vi "ELVIS III v1.0 Write PWM.vi"(8 "error in (no error)":errorcluster, 9 "PWM Configuration In":T1, 10 "Channel":T2, 11 "myRIO Ref In":T3) -> (0 "error out":errorcluster, 2 "PWM Configuration Out":T1, 3 "myRIO Ref Out":T3)   [LabVIEW 2021]
uses:
  <vilib>/myRIO/Common/Instrument Driver Framework/Utilities/typedefs/myRIO v1.0 Reference.ctl
  <vilib>/myRIO/Common/Instrument Driver Framework/Utilities/typedefs/Generic FPGA Reference.ctl
  <vilib>/myRIO/Common/Instrument Driver Framework/myRIO v1.0/PWM/typedefs/PWM Channels Enum.ctl
  <vilib>/myRIO/Common/Instrument Driver Framework/myRIO v1.0/PWM/typedefs/PWM Configuration v1.0.ctl
  <vilib>/myRIO/Common/Instrument Driver Framework/ELVIS III v1.0/PWM/typedefs/ELVIS III PWM Channels FPGA Reference.ctl
  <vilib>/myRIO/Common/Instrument Driver Framework/Utilities/vis/Calculate Clock Settings.vi
  <vilib>/myRIO/Common/Instrument Driver Framework/Utilities/vis/Calculate TOP (Phase Correct Mode).vi
  <vilib>/myRIO/Common/Instrument Driver Framework/Utilities/vis/Calculate TOP (Normal Mode).vi
  <vilib>/myRIO/Common/Instrument Driver Framework/Utilities/vis/Calculate Frequency (Phase Correct Mode).vi
  <vilib>/myRIO/Common/Instrument Driver Framework/Utilities/vis/Calculate Frequency (Normal Mode).vi
  <vilib>/rvi/errors/niLvFpgaAdjustHostInterfaceError.vi
  <vilib>/rvi/interface/nirviReadWriteControl/nirviReadWriteControl.xnode
  NiFpgaLv.dll
  <vilib>/rvi/interface/Simulation/niFpgaSimulationCallBeginRW.vi
panel:
  # "This VI writes a value to each output compare register (OCCRA and OCCRB) for a particular PWM channel. The output compare values are used to define the duty cycles of the PWM outputs. Please see Block Diagram for details."
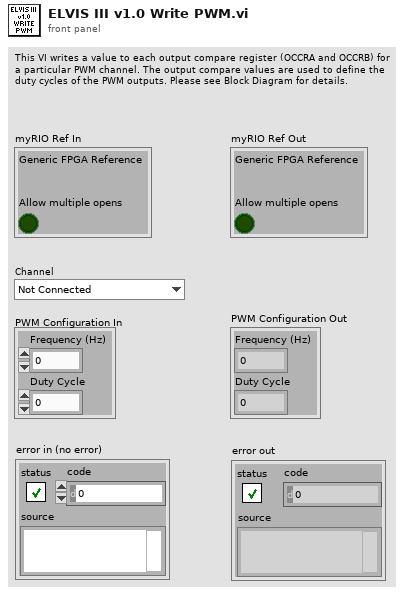
[diagram p1: front panel]
types:
  T1 = typedef "PWM Configuration v1.0.ctl" = cluster{"Frequency (Hz)":dbl, "Duty Cycle":dbl}
  T2 = typedef "PWM Channels Enum.ctl" = enum16{"Not Connected", "C/PWM0", "C/PWM1", "A/PWM0", "A/PWM1", "A/PWM2", "A/PWM3", "A/PWM4", "A/PWM5", "A/PWM6", "A/PWM7", "A/PWM8", "A/PWM9", "A/PWM10", "A/PWM11", "A/PWM12", "A/PWM13", "A/PWM14", "A/PWM15", "A/PWM16", "A/PWM17", "A/PWM18", "A/PWM19", "B/PWM0", "B/PWM1", "B/PWM2", "B/PWM3", "B/PWM4", "B/PWM5", "B/PWM6", "B/PWM7", "B/PWM8", "B/PWM9", "B/PWM10", "B/PWM11", "B/PWM12", "B/PWM13", "B/PWM14", "B/PWM15", "B/PWM16", "B/PWM17", "B/PWM18", "B/PWM19", "PWM/PWM0", "PWM/PWM1", "PWM/PWM2", "PWM/PWM3", "PWM/PWM4", "PWM/PWM5", "PWM/PWM6", "PWM/PWM7", "PWM/PWM8", "PWM/PWM9"}
  T3 = typedef "myRIO v1.0 Reference.ctl" = cluster{"Generic FPGA Reference":T4, "Allow multiple opens":bool}
  T4 = typedef "Generic FPGA Reference.ctl" = refnum<k20>
  T5 = typedef "ELVIS III PWM Channels FPGA Reference.ctl" = refnum<k20>
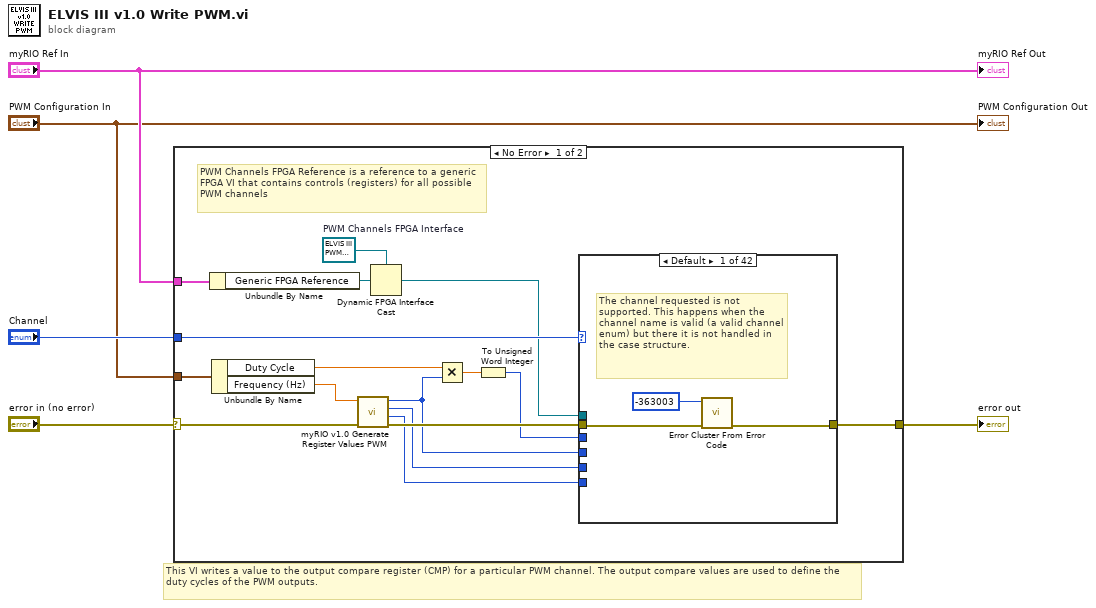
[diagram p0: block diagram]
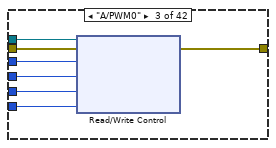
[diagram p3: hidden frame]
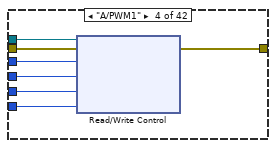
[diagram p4: hidden frame]
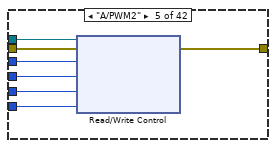
[diagram p5: hidden frame]
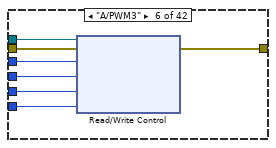
[diagram p6: hidden frame]
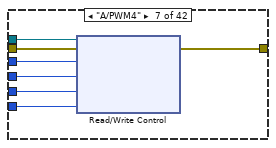
[diagram p7: hidden frame]
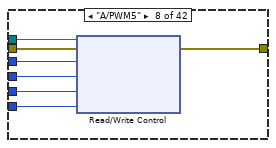
[diagram p8: hidden frame]
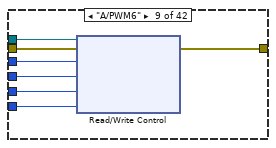
[diagram p9: hidden frame]
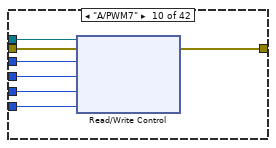
[diagram p10: hidden frame]
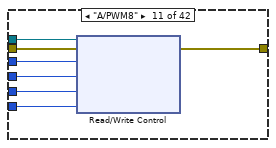
[diagram p11: hidden frame]
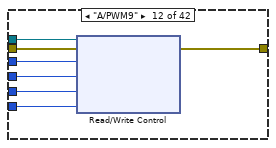
[diagram p12: hidden frame]
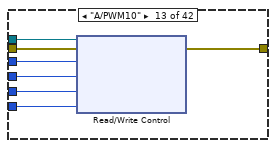
[diagram p13: hidden frame]
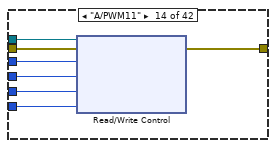
[diagram p14: hidden frame]
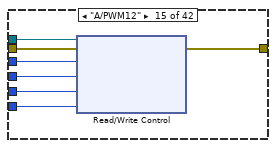
[diagram p15: hidden frame]
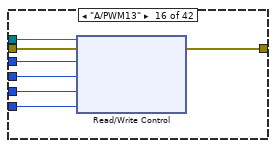
[diagram p16: hidden frame]
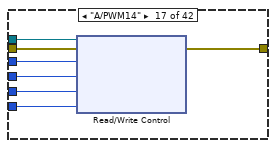
[diagram p17: hidden frame]
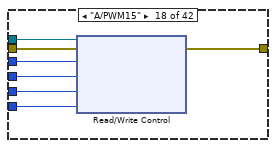
[diagram p18: hidden frame]
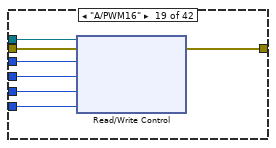
[diagram p19: hidden frame]
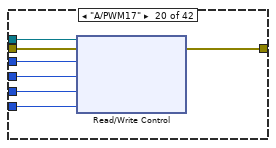
[diagram p20: hidden frame]
diagram:
  # "This VI writes a value to the output compare register (CMP) for a particular PWM channel. The output compare values are used to define the duty cycles of the PWM outputs."
  n1 = case shown="No Error" "error in (no error)" {
    selector: "error in (no error)" -> [w16 w306]
    tunnel: "myRIO Ref In" -> [w20 _]
    tunnel: [w6 w306] -> w4
    tunnel: "Channel" -> [w13 _]
    tunnel: "PWM Configuration In" -> [w15 _]
    frame No Error {
      w21 = T5 refnum  # PWM Channels FPGA Interface
      # "PWM Channels FPGA Reference is a reference to a generic FPGA VI that contains controls (registers) for all possible PWM channels"
      n2 = Unbundle By Name(w20) -> ("Generic FPGA Reference"=w19:T4)
      n3 = Unbundle By Name(w15) -> ("Duty Cycle"=w18:dbl, "Frequency (Hz)"=w14:dbl)
      n4 = call <vilib>:"myRIO v1.0 Generate Register Values PWM.vi"("error in (no error)"=w16, "Frequency (Hz)"=w14) -> ("error out"=w11:errorcluster, "PWM.CS"=w7:u8, "PWM.CNFG"=w8:u8, "PWM.MAX"=w9:u16)  [unwired: 5 in, 1 out]
      n5 = Dynamic FPGA Interface Cast(Session In=w21, Type=w19) -> (Session Out=w12:T5)
      n6 = Multiply(x=w18, y=w9) -> (x*y=w17:dbl)
      n7 = To Unsigned Word Integer(number=w17) -> (unsigned 16bit integer=w10:u16)
      n8 = case shown="Default" w13 {
        tunnel: w12 -> [_ _ w32 w39 w46 w53 w60 w67 w74 w81 w88 w95 w102 w109 w116 w123 w130 w137 w144 w151 w158 w165 w172 w179 w186 w193 w200 w207 w214 w221 w228 w235 w242 w249 w256 w263 w270 w277 w284 w291 w298 w305]
        tunnel: w11 -> [w23 w25 w31 w38 w45 w52 w59 w66 w73 w80 w87 w94 w101 w108 w115 w122 w129 w136 w143 w150 w157 w164 w171 w178 w185 w192 w199 w206 w213 w220 w227 w234 w241 w248 w255 w262 w269 w276 w283 w290 w297 w304]
        tunnel: w10 -> [_ _ w30 w37 w44 w51 w58 w65 w72 w79 w86 w93 w100 w107 w114 w121 w128 w135 w142 w149 w156 w163 w170 w177 w184 w191 w198 w205 w212 w219 w226 w233 w240 w247 w254 w261 w268 w275 w282 w289 w296 w303]
        tunnel: w9 -> [_ _ w29 w36 w43 w50 w57 w64 w71 w78 w85 w92 w99 w106 w113 w120 w127 w134 w141 w148 w155 w162 w169 w176 w183 w190 w197 w204 w211 w218 w225 w232 w239 w246 w253 w260 w267 w274 w281 w288 w295 w302]
        tunnel: w8 -> [_ _ w28 w35 w42 w49 w56 w63 w70 w77 w84 w91 w98 w105 w112 w119 w126 w133 w140 w147 w154 w161 w168 w175 w182 w189 w196 w203 w210 w217 w224 w231 w238 w245 w252 w259 w266 w273 w280 w287 w294 w301]
        tunnel: w7 -> [_ _ w27 w34 w41 w48 w55 w62 w69 w76 w83 w90 w97 w104 w111 w118 w125 w132 w139 w146 w153 w160 w167 w174 w181 w188 w195 w202 w209 w216 w223 w230 w237 w244 w251 w258 w265 w272 w279 w286 w293 w300]
        tunnel: [w22 w25 w26 w33 w40 w47 w54 w61 w68 w75 w82 w89 w96 w103 w110 w117 w124 w131 w138 w145 w152 w159 w166 w173 w180 w187 w194 w201 w208 w215 w222 w229 w236 w243 w250 w257 w264 w271 w278 w285 w292 w299] -> w6
        frame Default {
          # "The channel requested is not supported. This happens when the channel name is valid (a valid channel enum) but there it is not handled in the case structure."
          n9 = call <vilib>:"Error Cluster From Error Code.vi"("error in (no error)"=w23, "error code (0)"=-363003) -> ("error out"=w22:errorcluster)  [unwired: 7 in]
        }
        frame "Not Connected" {
        }
        frame "A/PWM0" {
          n10 = xnode "Read/Write Control"("FPGA VI Reference In"=w32, "error in"=w31, "PWM.A_0.CMP"=w30, "PWM.A_0.MAX"=w29, "PWM.A_0.CNFG"=w28, "PWM.A_0.CS"=w27) -> ("error out"=w26:errorcluster)  [unwired: 1 out]
        }
        frame "A/PWM1" {
          n11 = xnode "Read/Write Control"("FPGA VI Reference In"=w39, "error in"=w38, "PWM.A_1.CMP"=w37, "PWM.A_1.MAX"=w36, "PWM.A_1.CNFG"=w35, "PWM.A_1.CS"=w34) -> ("error out"=w33:errorcluster)  [unwired: 1 out]
        }
        frame "A/PWM2" {
          n12 = xnode "Read/Write Control"("FPGA VI Reference In"=w46, "error in"=w45, "PWM.A_2.CMP"=w44, "PWM.A_2.MAX"=w43, "PWM.A_2.CNFG"=w42, "PWM.A_2.CS"=w41) -> ("error out"=w40:errorcluster)  [unwired: 1 out]
        }
        frame "A/PWM3" {
          n13 = xnode "Read/Write Control"("FPGA VI Reference In"=w53, "error in"=w52, "PWM.A_3.CMP"=w51, "PWM.A_3.MAX"=w50, "PWM.A_3.CNFG"=w49, "PWM.A_3.CS"=w48) -> ("error out"=w47:errorcluster)  [unwired: 1 out]
        }
        frame "A/PWM4" {
          n14 = xnode "Read/Write Control"("FPGA VI Reference In"=w60, "error in"=w59, "PWM.A_4.CMP"=w58, "PWM.A_4.MAX"=w57, "PWM.A_4.CNFG"=w56, "PWM.A_4.CS"=w55) -> ("error out"=w54:errorcluster)  [unwired: 1 out]
        }
        frame "A/PWM5" {
          n15 = xnode "Read/Write Control"("FPGA VI Reference In"=w67, "error in"=w66, "PWM.A_5.CMP"=w65, "PWM.A_5.MAX"=w64, "PWM.A_5.CNFG"=w63, "PWM.A_5.CS"=w62) -> ("error out"=w61:errorcluster)  [unwired: 1 out]
        }
        frame "A/PWM6" {
          n16 = xnode "Read/Write Control"("FPGA VI Reference In"=w74, "error in"=w73, "PWM.A_6.CMP"=w72, "PWM.A_6.MAX"=w71, "PWM.A_6.CNFG"=w70, "PWM.A_6.CS"=w69) -> ("error out"=w68:errorcluster)  [unwired: 1 out]
        }
        frame "A/PWM7" {
          n17 = xnode "Read/Write Control"("FPGA VI Reference In"=w81, "error in"=w80, "PWM.A_7.CMP"=w79, "PWM.A_7.MAX"=w78, "PWM.A_7.CNFG"=w77, "PWM.A_7.CS"=w76) -> ("error out"=w75:errorcluster)  [unwired: 1 out]
        }
        frame "A/PWM8" {
          n18 = xnode "Read/Write Control"("FPGA VI Reference In"=w88, "error in"=w87, "PWM.A_8.CMP"=w86, "PWM.A_8.MAX"=w85, "PWM.A_8.CNFG"=w84, "PWM.A_8.CS"=w83) -> ("error out"=w82:errorcluster)  [unwired: 1 out]
        }
        frame "A/PWM9" {
          n19 = xnode "Read/Write Control"("FPGA VI Reference In"=w95, "error in"=w94, "PWM.A_9.CMP"=w93, "PWM.A_9.MAX"=w92, "PWM.A_9.CNFG"=w91, "PWM.A_9.CS"=w90) -> ("error out"=w89:errorcluster)  [unwired: 1 out]
        }
        frame "A/PWM10" {
          n20 = xnode "Read/Write Control"("FPGA VI Reference In"=w102, "error in"=w101, "PWM.A_10.CMP"=w100, "PWM.A_10.MAX"=w99, "PWM.A_10.CNFG"=w98, "PWM.A_10.CS"=w97) -> ("error out"=w96:errorcluster)  [unwired: 1 out]
        }
        frame "A/PWM11" {
          n21 = xnode "Read/Write Control"("FPGA VI Reference In"=w109, "error in"=w108, "PWM.A_11.CMP"=w107, "PWM.A_11.MAX"=w106, "PWM.A_11.CNFG"=w105, "PWM.A_11.CS"=w104) -> ("error out"=w103:errorcluster)  [unwired: 1 out]
        }
        frame "A/PWM12" {
          n22 = xnode "Read/Write Control"("FPGA VI Reference In"=w116, "error in"=w115, "PWM.A_12.CMP"=w114, "PWM.A_12.MAX"=w113, "PWM.A_12.CNFG"=w112, "PWM.A_12.CS"=w111) -> ("error out"=w110:errorcluster)  [unwired: 1 out]
        }
        frame "A/PWM13" {
          n23 = xnode "Read/Write Control"("FPGA VI Reference In"=w123, "error in"=w122, "PWM.A_13.CMP"=w121, "PWM.A_13.MAX"=w120, "PWM.A_13.CNFG"=w119, "PWM.A_13.CS"=w118) -> ("error out"=w117:errorcluster)  [unwired: 1 out]
        }
        frame "A/PWM14" {
          n24 = xnode "Read/Write Control"("FPGA VI Reference In"=w130, "error in"=w129, "PWM.A_14.CMP"=w128, "PWM.A_14.MAX"=w127, "PWM.A_14.CNFG"=w126, "PWM.A_14.CS"=w125) -> ("error out"=w124:errorcluster)  [unwired: 1 out]
        }
        frame "A/PWM15" {
          n25 = xnode "Read/Write Control"("FPGA VI Reference In"=w137, "error in"=w136, "PWM.A_15.CMP"=w135, "PWM.A_15.MAX"=w134, "PWM.A_15.CNFG"=w133, "PWM.A_15.CS"=w132) -> ("error out"=w131:errorcluster)  [unwired: 1 out]
        }
        frame "A/PWM16" {
          n26 = xnode "Read/Write Control"("FPGA VI Reference In"=w144, "error in"=w143, "PWM.A_16.CMP"=w142, "PWM.A_16.MAX"=w141, "PWM.A_16.CNFG"=w140, "PWM.A_16.CS"=w139) -> ("error out"=w138:errorcluster)  [unwired: 1 out]
        }
        frame "A/PWM17" {
          n27 = xnode "Read/Write Control"("FPGA VI Reference In"=w151, "error in"=w150, "PWM.A_17.CMP"=w149, "PWM.A_17.MAX"=w148, "PWM.A_17.CNFG"=w147, "PWM.A_17.CS"=w146) -> ("error out"=w145:errorcluster)  [unwired: 1 out]
        }
        frame "A/PWM18" {
          n28 = xnode "Read/Write Control"("FPGA VI Reference In"=w158, "error in"=w157, "PWM.A_18.CMP"=w156, "PWM.A_18.MAX"=w155, "PWM.A_18.CNFG"=w154, "PWM.A_18.CS"=w153) -> ("error out"=w152:errorcluster)  [unwired: 1 out]
        }
        frame "A/PWM19" {
          n29 = xnode "Read/Write Control"("FPGA VI Reference In"=w165, "error in"=w164, "PWM.A_19.CMP"=w163, "PWM.A_19.MAX"=w162, "PWM.A_19.CNFG"=w161, "PWM.A_19.CS"=w160) -> ("error out"=w159:errorcluster)  [unwired: 1 out]
        }
        frame "B/PWM0" {
          n30 = xnode "Read/Write Control"("FPGA VI Reference In"=w172, "error in"=w171, "PWM.B_0.CMP"=w170, "PWM.B_0.MAX"=w169, "PWM.B_0.CNFG"=w168, "PWM.B_0.CS"=w167) -> ("error out"=w166:errorcluster)  [unwired: 1 out]
        }
        frame "B/PWM1" {
          n31 = xnode "Read/Write Control"("FPGA VI Reference In"=w179, "error in"=w178, "PWM.B_1.CMP"=w177, "PWM.B_1.MAX"=w176, "PWM.B_1.CNFG"=w175, "PWM.B_1.CS"=w174) -> ("error out"=w173:errorcluster)  [unwired: 1 out]
        }
        frame "B/PWM2" {
          n32 = xnode "Read/Write Control"("FPGA VI Reference In"=w186, "error in"=w185, "PWM.B_2.CMP"=w184, "PWM.B_2.MAX"=w183, "PWM.B_2.CNFG"=w182, "PWM.B_2.CS"=w181) -> ("error out"=w180:errorcluster)  [unwired: 1 out]
        }
        frame "B/PWM3" {
          n33 = xnode "Read/Write Control"("FPGA VI Reference In"=w193, "error in"=w192, "PWM.B_3.CMP"=w191, "PWM.B_3.MAX"=w190, "PWM.B_3.CNFG"=w189, "PWM.B_3.CS"=w188) -> ("error out"=w187:errorcluster)  [unwired: 1 out]
        }
        frame "B/PWM4" {
          n34 = xnode "Read/Write Control"("FPGA VI Reference In"=w200, "error in"=w199, "PWM.B_4.CMP"=w198, "PWM.B_4.MAX"=w197, "PWM.B_4.CNFG"=w196, "PWM.B_4.CS"=w195) -> ("error out"=w194:errorcluster)  [unwired: 1 out]
        }
        frame "B/PWM5" {
          n35 = xnode "Read/Write Control"("FPGA VI Reference In"=w207, "error in"=w206, "PWM.B_5.CMP"=w205, "PWM.B_5.MAX"=w204, "PWM.B_5.CNFG"=w203, "PWM.B_5.CS"=w202) -> ("error out"=w201:errorcluster)  [unwired: 1 out]
        }
        frame "B/PWM6" {
          n36 = xnode "Read/Write Control"("FPGA VI Reference In"=w214, "error in"=w213, "PWM.B_6.CMP"=w212, "PWM.B_6.MAX"=w211, "PWM.B_6.CNFG"=w210, "PWM.B_6.CS"=w209) -> ("error out"=w208:errorcluster)  [unwired: 1 out]
        }
        frame "B/PWM7" {
          n37 = xnode "Read/Write Control"("FPGA VI Reference In"=w221, "error in"=w220, "PWM.B_7.CMP"=w219, "PWM.B_7.MAX"=w218, "PWM.B_7.CNFG"=w217, "PWM.B_7.CS"=w216) -> ("error out"=w215:errorcluster)  [unwired: 1 out]
        }
        frame "B/PWM8" {
          n38 = xnode "Read/Write Control"("FPGA VI Reference In"=w228, "error in"=w227, "PWM.B_8.CMP"=w226, "PWM.B_8.MAX"=w225, "PWM.B_8.CNFG"=w224, "PWM.B_8.CS"=w223) -> ("error out"=w222:errorcluster)  [unwired: 1 out]
        }
        frame "B/PWM9" {
          n39 = xnode "Read/Write Control"("FPGA VI Reference In"=w235, "error in"=w234, "PWM.B_9.CMP"=w233, "PWM.B_9.MAX"=w232, "PWM.B_9.CNFG"=w231, "PWM.B_9.CS"=w230) -> ("error out"=w229:errorcluster)  [unwired: 1 out]
        }
        frame "B/PWM10" {
          n40 = xnode "Read/Write Control"("FPGA VI Reference In"=w242, "error in"=w241, "PWM.B_10.CMP"=w240, "PWM.B_10.MAX"=w239, "PWM.B_10.CNFG"=w238, "PWM.B_10.CS"=w237) -> ("error out"=w236:errorcluster)  [unwired: 1 out]
        }
        frame "B/PWM11" {
          n41 = xnode "Read/Write Control"("FPGA VI Reference In"=w249, "error in"=w248, "PWM.B_11.CMP"=w247, "PWM.B_11.MAX"=w246, "PWM.B_11.CNFG"=w245, "PWM.B_11.CS"=w244) -> ("error out"=w243:errorcluster)  [unwired: 1 out]
        }
        frame "B/PWM12" {
          n42 = xnode "Read/Write Control"("FPGA VI Reference In"=w256, "error in"=w255, "PWM.B_12.CMP"=w254, "PWM.B_12.MAX"=w253, "PWM.B_12.CNFG"=w252, "PWM.B_12.CS"=w251) -> ("error out"=w250:errorcluster)  [unwired: 1 out]
        }
        frame "B/PWM13" {
          n43 = xnode "Read/Write Control"("FPGA VI Reference In"=w263, "error in"=w262, "PWM.B_13.CMP"=w261, "PWM.B_13.MAX"=w260, "PWM.B_13.CNFG"=w259, "PWM.B_13.CS"=w258) -> ("error out"=w257:errorcluster)  [unwired: 1 out]
        }
        frame "B/PWM14" {
          n44 = xnode "Read/Write Control"("FPGA VI Reference In"=w270, "error in"=w269, "PWM.B_14.CMP"=w268, "PWM.B_14.MAX"=w267, "PWM.B_14.CNFG"=w266, "PWM.B_14.CS"=w265) -> ("error out"=w264:errorcluster)  [unwired: 1 out]
        }
        frame "B/PWM15" {
          n45 = xnode "Read/Write Control"("FPGA VI Reference In"=w277, "error in"=w276, "PWM.B_15.CMP"=w275, "PWM.B_15.MAX"=w274, "PWM.B_15.CNFG"=w273, "PWM.B_15.CS"=w272) -> ("error out"=w271:errorcluster)  [unwired: 1 out]
        }
        frame "B/PWM16" {
          n46 = xnode "Read/Write Control"("FPGA VI Reference In"=w284, "error in"=w283, "PWM.B_16.CMP"=w282, "PWM.B_16.MAX"=w281, "PWM.B_16.CNFG"=w280, "PWM.B_16.CS"=w279) -> ("error out"=w278:errorcluster)  [unwired: 1 out]
        }
        frame "B/PWM17" {
          n47 = xnode "Read/Write Control"("FPGA VI Reference In"=w291, "error in"=w290, "PWM.B_17.CMP"=w289, "PWM.B_17.MAX"=w288, "PWM.B_17.CNFG"=w287, "PWM.B_17.CS"=w286) -> ("error out"=w285:errorcluster)  [unwired: 1 out]
        }
        frame "B/PWM18" {
          n48 = xnode "Read/Write Control"("FPGA VI Reference In"=w298, "error in"=w297, "PWM.B_18.CMP"=w296, "PWM.B_18.MAX"=w295, "PWM.B_18.CNFG"=w294, "PWM.B_18.CS"=w293) -> ("error out"=w292:errorcluster)  [unwired: 1 out]
        }
        frame "B/PWM19" {
          n49 = xnode "Read/Write Control"("FPGA VI Reference In"=w305, "error in"=w304, "PWM.B_19.CMP"=w303, "PWM.B_19.MAX"=w302, "PWM.B_19.CNFG"=w301, "PWM.B_19.CS"=w300) -> ("error out"=w299:errorcluster)  [unwired: 1 out]
        }
      }
    }
    frame Error {
      # "Nothing to do since there was an incoming error."
    }
  }
  "error out" <- w4
  "myRIO Ref Out" <- "myRIO Ref In"
  "PWM Configuration Out" <- "PWM Configuration In"
